vi "Stop Core.vi"(10 "final error code":i32, 11 "DAQ Actor in":refnum<class "DAQ Actor.lvclass">) -> (3 "DAQ Actor out":refnum<class "DAQ Actor.lvclass">)   [LabVIEW 2012, in "Data Acquisition.lvlib" / "DAQ Actor.lvclass"]
doc: "(<B>Filename</B>: Actor Framework.lvlib:Actor.lvclass:Stop Core.vi)\n\nDefines what the actor does before it stops. Use the <B>final error code</B> input to determine whether the actor shut down in response to an error.\n\nBy default, this method does nothing. A descendant class may override it to define behavior, such as shutting down any processes the actor initiated in its override of the Actor Core method."
uses:
  DAQ Actor.lvclass
  <vilib>/ActorFramework/Actor/Actor.lvclass
  DAQ Actor.lvclass/DAQ Actor.ctl
  TCP Server/TCP Writer Messages/Delete Wfm Header Msg/Delete Wfm Header Msg.lvclass/Delete Wfm Header Msg.ctl
  <vilib>/ActorFramework/Message Enqueuer/Message Enqueuer.lvclass/Message Enqueuer.ctl
  <vilib>/ActorFramework/Message Enqueuer/Enqueue.vi
  <vilib>/ActorFramework/Message Priority Queue/Priority Enqueue.vi
  TCP Server/TCP Writer Messages/Delete Wfm Header Msg/Delete Wfm Header Msg.lvclass
  Class DAQ Task/DAQ Task.lvclass
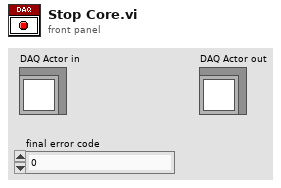
[diagram p1: front panel]
types:
  T1 = typedef "TE_Designator.ctl" = enum16{"High Speed", "Low Speed"}
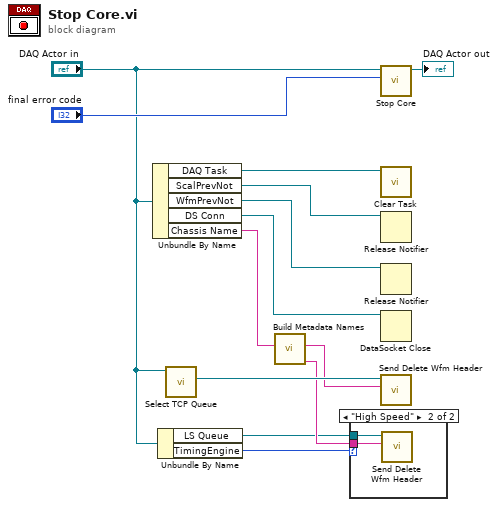
[diagram p0: block diagram]
diagram:
  n1 = Unbundle By Name("DAQ Actor in") -> ("DAQ Task"=w8:refnum<class "DAQ Task.lvclass">, "ScalPrevNot"=w11:refnum<notifier>, "WfmPrevNot"=w10:refnum<notifier>, "DS Conn"=w9:refnum<k13>, "Chassis Name"=w6:string)
  n2 = Unbundle By Name("DAQ Actor in") -> ("LS Queue"=w2:refnum<class "Message Enqueuer.lvclass">, "TimingEngine"=w1:T1)
  n3 = call "Select TCP Queue.vi"("DAQ Actor in"="DAQ Actor in") -> ("TCP Queue"=w7:refnum<class "Message Enqueuer.lvclass">)  [unwired: 8 in, 2 out]
  n4 = call "Build Metadata Names.vi"("Chassis Name"=w6) -> ("Modbus Wfm Hdr"=w4:string, "Wfm Hdr"=w5:string)  [unwired: 6 in, 3 out]
  n5 = case shown="\"High Speed\"" w1 {
    tunnel: w4 -> [_ w15]
    tunnel: w2 -> [_ w14]
    frame "Low Speed" {
    }
    frame "High Speed" {
      n6 = call "Send Delete Wfm Header.vi"("Metadata"=w15, "Message Enqueuer"=w14) -> ()  [unwired: 8 in, 2 out]
    }
  }
  n7 = call-parent "Stop Core.vi"("final error code"="final error code", "Actor in"="DAQ Actor in") -> ("Actor out"=→"DAQ Actor out":refnum<class "DAQ Actor.lvclass">)  [unwired: 9 in]
  n8 = call "Clear Task.vi"("DAQ Task in"=w8) -> ()  [unwired: 9 in, 2 out]
  n9 = Release Notifier(notifier=w11) -> ()  [unwired: 2 in, 3 out]
  n10 = Release Notifier(notifier=w10) -> ()  [unwired: 2 in, 3 out]
  n11 = DataSocket Close(11:w9) -> ()  [unwired: 2 in, 2 out]
  n12 = call "Send Delete Wfm Header.vi"("Metadata"=w5, "Message Enqueuer"=w7) -> ()  [unwired: 8 in, 2 out]
